vi "getPayloadRequirement.vi"(11 "SUBSCRIBE in":refnum<class "SUBSCRIBE.lvclass">) -> (2 "Requirement":T1, 3 "SUBSCRIBE out":refnum<class "SUBSCRIBE.lvclass">)   [LabVIEW 2013, in "MQTT_Control_Packets.lvlib" / "SUBSCRIBE.lvclass"]
uses:
  SUBSCRIBE.lvclass
  ControlPacket/Requirement -- enum.ctl
  ControlPacket/ControlPacket.lvclass
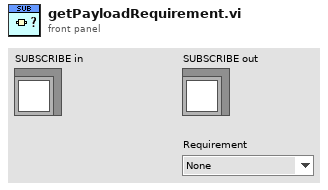
[diagram p1: front panel]
types:
  T1 = typedef "MQTT_Control_Packets.lvlib/ControlPacket.lvclass/Requirement -- enum.ctl" = enum16{"None", "Optional", "Required"}
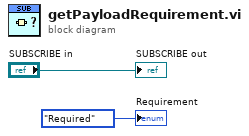
[diagram p0: block diagram]
diagram:
  "SUBSCRIBE out" <- "SUBSCRIBE in"
  "Requirement" <- Requirement_--_enum."Required" ("Requirement")
